vi "HP53220 Measure FrequencyOF24.vi"(1 "GPIB Bus":i32 min=0 max=5, 3 "Number of Readings":i32=1 min=1, 4 "error in":errorcluster, 5 "GPIB Address":i16=3 max=31, 6 "Gate Time":dbl=1.0 min=0.0 max=1000.0 step=0.1 format="%.2f", 7 "Channel(1,2,3)":enum16{"Channel 1", "Channel 2", "Channel 3"}(ring)) -> (0 "error out":errorcluster, 2 "Frequency":dbl format="%.6f")   [LabVIEW 2024]
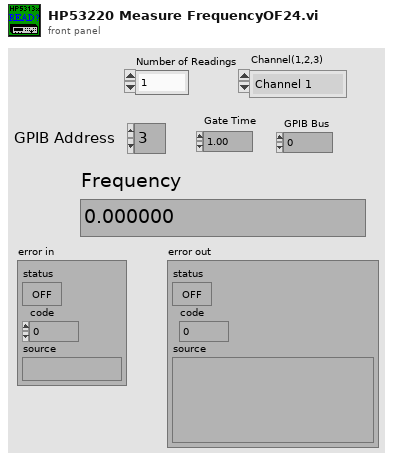
[diagram p1: front panel]
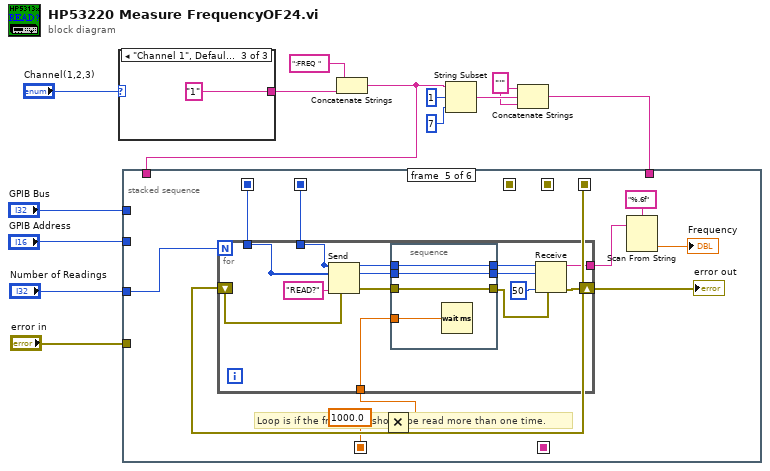
[diagram p0: block diagram]
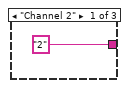
[diagram p2: hidden frame]
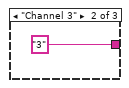
[diagram p3: hidden frame]
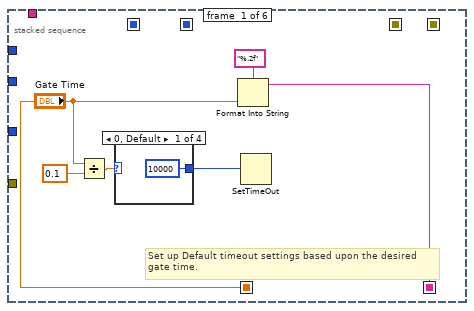
[diagram p4: hidden frame]
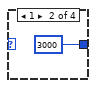
[diagram p5: hidden frame]
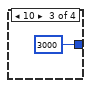
[diagram p6: hidden frame]
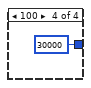
[diagram p7: hidden frame]
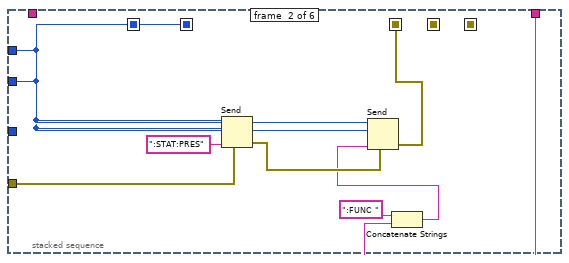
[diagram p8: hidden frame]
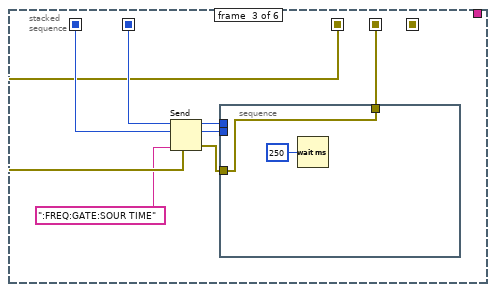
[diagram p9: hidden frame]
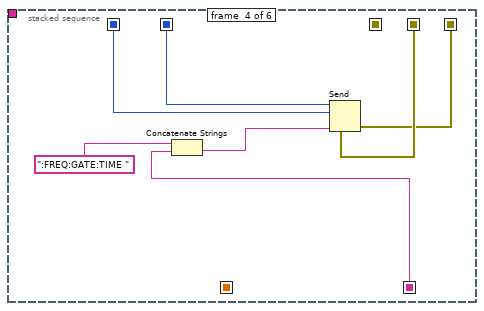
[diagram p10: hidden frame]
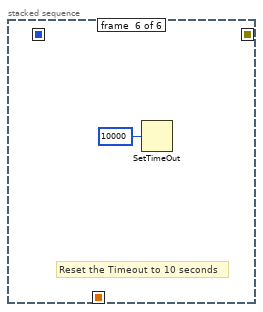
[diagram p11: hidden frame]
diagram:
  w4 = "'"
  n1 = case shown="\"Channel 1\", Default" "Channel(1,2,3)" {
    tunnel: ["2" "3" "1"] -> w10
    frame "Channel 2" {
    }
    frame "Channel 3" {
    }
    frame "Channel 1", Default {
    }
  }
  n2 = Concatenate Strings(":FREQ ", w10) -> (w8:string)
  n3 = String Subset(string=w8, offset (0)=1, length (rest)=7 ("length (rest)")) -> (substring=w5:string)
  n4 = Concatenate Strings(w4, w5, w4) -> (w3:string)
  n5 = stacked-sequence {
    seq-local: [_ w28 _ _ _ _] -> [_ _ w40 w50 w55 _]
    seq-local: [w21 _ _ _ _ _] -> [_ _ _ w48 _ _]
    seq-local: [_ w29 _ _ _ _] -> [_ _ w41 w47 w56 _]
    seq-local: [_ w34 _ _ _ _] -> [_ _ w39 _ _ _]
    seq-local: [_ _ w37 _ _ _] -> [_ _ _ w46 _ _]
    seq-local: [_ _ _ w45 _ _] -> [_ _ _ _ w58 _]
    seq-local: ["Gate Time" _ _ _ _ _] -> [_ _ _ _ w53 _]
    tunnel: "GPIB Address" -> [_ w28 _ _ _ _]
    tunnel: "GPIB Bus" -> [_ w29 _ _ _ _]
    tunnel: w8 -> [_ _ _ _ _ _]
    tunnel: w3 -> [_ w30 _ _ _ _]
    tunnel: "error in" -> [_ w27 _ _ _ _]
    tunnel: "Number of Readings" -> [_ _ _ _ w57 _]
    frame #0 {
      # "Set up Default timeout settings based upon the desired \ngate time."
      n6 = Divide(x="Gate Time", y=0.1) -> (x/y=w19:dbl)
      n7 = case shown="0, Default" w19 {
        tunnel: [10000 3000 3000 30000] -> w20
        frame 0, Default {
        }
        frame 1 {
        }
        frame 10 {
        }
        frame 100 {
        }
      }
      n8 = Format Into String(format string="%.2f" ("Format String"), "Gate Time") -> (resulting string=w21:string)  [unwired: 2 in, 1 out]
      n9 = SetTimeOut(1:w20) -> ()  [unwired: 1 out]
    }
    frame #1 {
      n10 = Send(0:w29, 2:w28, 4:w27, 5:":STAT:PRES" ("data string")) -> (8:w33:errorcluster)  [unwired: 1 in, 2 out]
      n11 = Concatenate Strings(":FUNC " ("data string"), w30) -> (w31:string)
      n12 = Send(0:w29, 2:w28, 4:w33, 5:w31) -> (8:w34:errorcluster)  [unwired: 1 in, 2 out]
    }
    frame #2 {
      n13 = Send(0:w41, 2:w40, 4:w39, 5:":FREQ:GATE:SOUR TIME" ("data string")) -> (8:w38:errorcluster)  [unwired: 1 in, 2 out]
      n14 = stacked-sequence {
        tunnel: w41 -> [_]
        tunnel: w40 -> [_]
        tunnel: w38 -> [w42]
        tunnel: [w42] -> w37
        frame #0 {
          n15 = Wait (ms)(milliseconds to wait=u32 250) -> ()  [unwired: 1 out]
        }
      }
    }
    frame #3 {
      n16 = Concatenate Strings(":FREQ:GATE:TIME " ("data string"), w48) -> (w49:string)
      n17 = Send(0:w47, 2:w50, 4:w46, 5:w49) -> (8:w45:errorcluster)  [unwired: 1 in, 2 out]
    }
    frame #4 {
      # "Loop is if the frequency should be read more than one time."
      n18 = Multiply(x=1000.0, y=w53) -> (x*y=w51:dbl)
      n19 = for {
        N: w57 -> [_]
        tunnel: w55 -> [w64]
        tunnel: w56 -> [w63]
        tunnel: [w72] -> w59
        shift-right: [w69] -> w54
        shift-left: w58 -> [w71]
        tunnel: w51 -> [w68]
        n20 = Send(0:w63, 2:w64, 4:w71, 5:"READ?" ("data string")) -> (8:w67:errorcluster)  [unwired: 1 in, 2 out]
        n21 = stacked-sequence {
          tunnel: w68 -> [w77]
          tunnel: w67 -> [w74]
          tunnel: [w75] -> w66
          tunnel: [w76] -> w65
          tunnel: w64 -> [w76]
          tunnel: w63 -> [w75]
          tunnel: [w74] -> w62
          frame #0 {
            n22 = Wait (ms)(milliseconds to wait=w77) -> ()  [unwired: 1 out]
          }
        }
        n23 = Receive(4:w62, 6:50 ("count"), 8:w65, 9:w66) -> (0:w69:errorcluster, 3:w72:string)  [unwired: 1 in, 2 out]
      }
      "error out" <- w54
      n24 = Scan From String(format string="%.6f" ("Format String"), input string=w59) -> (output 1=→"Frequency":dbl)  [unwired: 3 in, 3 out]
    }
    frame #5 {
      # "Reset the Timeout to 10 seconds"
      n25 = SetTimeOut(1:10000 ("new timeout (10000)")) -> ()  [unwired: 1 out]
    }
  }
